vi "MFC W HCC2.vi"(8 "error in":errorcluster, 10 "Byte array":u8[](array[numeric])=[76, 48, 48, 48, 48, 48, 13]) -> (0 "error out":errorcluster)   [LabVIEW 2014]
uses:
  <vilib>/rvi/eio/common/nirviEmuTemplateMethod_errors.vi
  <vilib>/eio/EIOMethodNode/EIOMethodNode.xnode
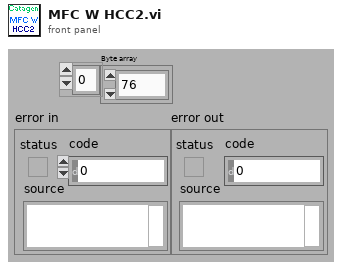
[diagram p1: front panel]
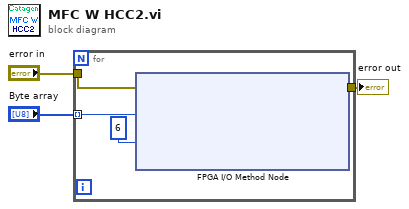
[diagram p0: block diagram]
diagram:
  n1 = for {
    tunnel: "Byte array" -> [w6] mode=indexing
    tunnel: [w5] -> w2
    tunnel: "error in" -> [w4]
    n2 = xnode "FPGA I/O Method Node"("error in"=w4, "Data"=w6, "Timeout (ms)"=6) -> ("error out"=w5:errorcluster)  [unwired: 1 in, 2 out]
  }
  "error out" <- w2
